vi "HSE Logger - UE Handler Quickstart.vi"   [LabVIEW 2024]
uses:
  <vilib>/Hampel Software Engineering/HSE Logger/LogLevel.ctl
  <vilib>/Hampel Software Engineering/HSE Logger/Handler/UserEventHandler/UserEventHandler.lvclass
  C:/Program Files (x86)/National Instruments/LabVIEW 2024/vi.lib/Hampel Software Engineering/HSE Logger/Handler/Handler.lvclass
  <vilib>/Hampel Software Engineering/HSE Logger/hse-logger.lvlib
types:
  T1 = typedef "hse-logger.lvlib/LogLevel.ctl" = enum16{"DEBUG", "INFO", "WARNING", "ERROR", "CRITICAL"}
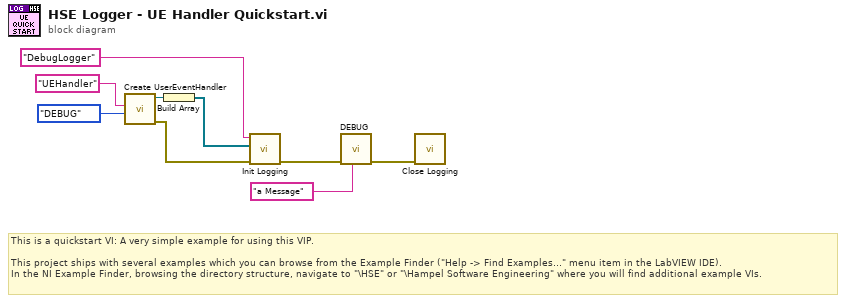
[diagram p0: block diagram]
diagram:
  # "This is a quickstart VI: A very simple example for using this VIP.\n\nThis project ships with several examples which you can browse from the Example Finder (\"Help -> Find Examples…\" menu item in the LabVIEW IDE).\nIn the NI Example Finder, browsing the directory structure, navigate to \"\\HSE\" or \"\\Hampel Software Engineering\" where you will find additional example VIs."
  n1 = call <vilib>:"Create UserEventHandler.vi"("Level"=LogLevel."DEBUG", "Name"="UEHandler") -> ("error out"=w9:errorcluster, "UserEventHandler out"=w6:refnum<class "UserEventHandler.lvclass">)  [unwired: 8 in]
  n2 = Build Array(w6) -> (w5:refnum<class "UserEventHandler.lvclass">[])
  n3 = call <vilib>:"Init Logging.vi"("error in"=w9, "Handlers"=w5, "Name"="DebugLogger") -> ("error out"=w8:errorcluster)  [unwired: 8 in]
  n4 = call <vilib>:"DEBUG.vi"("Message"="a Message", "error in"=w8) -> ("error out"=w7:errorcluster)  [unwired: 9 in]
  n5 = call <vilib>:"Close Logging.vi"("error in"=w7) -> ()  [unwired: 10 in, 1 out]
